vi "Handle Error.vi"(8 "error in (no error)":errorcluster, 11 "UI in":refnum<class "UI.lvclass">) -> (0 "error out":errorcluster, 2 "stop actor?":bool=TRUE, 3 "UI out":refnum<class "UI.lvclass">)   [LabVIEW 2016, in "Generic UI Actor.lvlib" / "UI.lvclass"]
doc: "(<B>Filename</B>: Actor Framework.lvlib:Actor.lvclass:Handle Error.vi)\n\nDefines how the actor handles an error that occurred while processing a message. By default, this method does nothing except stop the actor."
uses:
  <userlib>/Common Components/User Interface/UI.lvclass
  C:/Program Files (x86)/National Instruments/LabVIEW 2016/vi.lib/ActorFramework/Actor/Actor.lvclass
  <vilib>/ActorFramework/Actor/Actor.lvclass/Actor.ctl
  <vilib>/ActorFramework/Message Enqueuer/Message Enqueuer.lvclass/Message Enqueuer.ctl
  <vilib>/ActorFramework/Message Enqueuer/Init from Existing Queue.vi
  <vilib>/ActorFramework/Message Enqueuer/Message Enqueuer.lvclass
  <vilib>/ActorFramework/Actor/Actor.lvclass
  <userlib>/Common Components/User Interface/Messages/Update Status Display/Update Status Display.lvclass
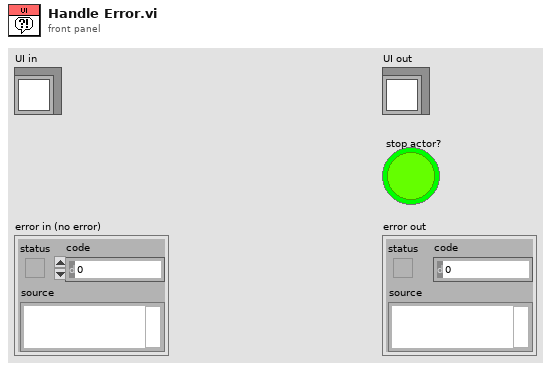
[diagram p1: front panel]
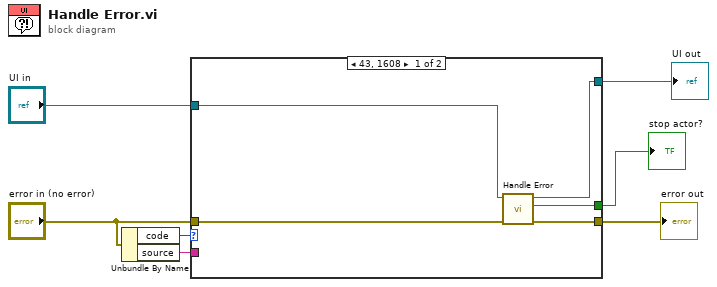
[diagram p0: block diagram]
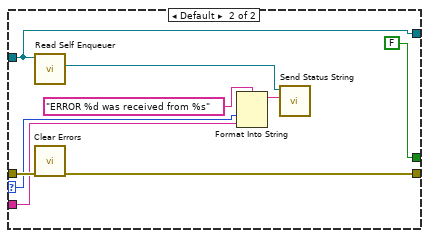
[diagram p2: hidden frame]
diagram:
  n1 = Unbundle By Name("error in (no error)") -> ("code"=w7:i32, "source"=w1:string)
  n2 = case shown="43, 1608" w7 {
    selector: w7 -> [_ w16]
    tunnel: "UI in" -> [w11 w14]
    tunnel: [w12 w14] -> w4
    tunnel: "error in (no error)" -> [w9 w21]
    tunnel: [w8 w20] -> w3
    tunnel: [w10 FALSE ("stop actor?")] -> w2
    tunnel: w1 -> [_ w17]
    frame 43, 1608 {
      n3 = call-parent "Handle Error.vi"("error in (no error)"=w9, "Actor in"=w11) -> ("error out"=w8:errorcluster, "stop actor?"=w10:bool, "Actor out"=w12:refnum<class "UI.lvclass">)  [unwired: 7 in]
    }
    frame Default {
      n4 = call <vilib>:"Read Self Enqueuer.vi"("Actor"=w14) -> ("Self Enqueuer"=w15:refnum<class "Message Enqueuer.lvclass">)  [unwired: 10 in]
      n5 = call <vilib>:"Clear Errors.vi"("error in (no error)"=w21) -> ("error out"=w20:errorcluster)  [unwired: 5 in, 1 out]
      n6 = Format Into String(format string="ERROR %d was received from %s", w16, w17) -> (resulting string=w13:string)  [unwired: 2 in, 1 out]
      n7 = call <userlib>:"Send Status String.vi"("String"=w13, "Message Enqueuer in"=w15) -> ()  [unwired: 8 in, 2 out]
    }
  }
  "UI out" <- w4
  "error out" <- w3
  "stop actor?" <- w2
